vi "(Old Driver) Block Write Iterator.vi"(8 "error in (no error)":errorcluster, 9 "Iterations (1000)":i32=110, 10 "Channel Count":i32, 11 "VMIC-5565":T1) -> (0 "error out":errorcluster, 1 "Histogram Graph":T2(graph), 2 "Metrics":T3 {"Transfer Rate" format="%.2pB/s"; "Duration Std. Dev." format="%.0f µs"; "Duration Average" format="%.0f µs"}, 3 "VMIC-5565 out":T1)   [LabVIEW 2016]
uses:
  Controls/Throughput Metrics.ctl
  <instrlib>/GE 5565 PIORC/Public/DMA Interrupt/GE5565 DMA Write Interrupt (U8) Cluster.vi
  <instrlib>/GE 5565 PIORC/GE 5565 PIORC.lvlib
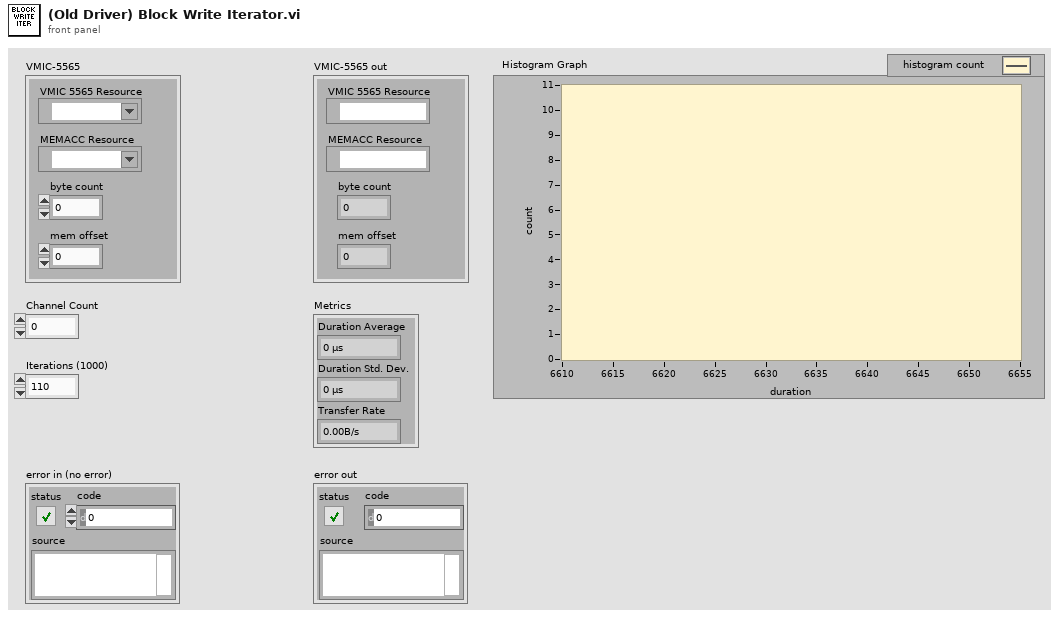
[diagram p1: front panel]
types:
  T1 = cluster{"VMIC 5565 Resource":refnum<visa-resource-name>, "MEMACC Resource":refnum<visa-resource-name>, "byte count":u32, "mem offset":u32}
  T2 = cluster{"X Values":dbl[], "Histogram: h(x)":i32[]}
  T3 = typedef "Throughput Metrics.ctl" = cluster{"Duration Average":u32, "Duration Std. Dev.":u32, "Transfer Rate":dbl}
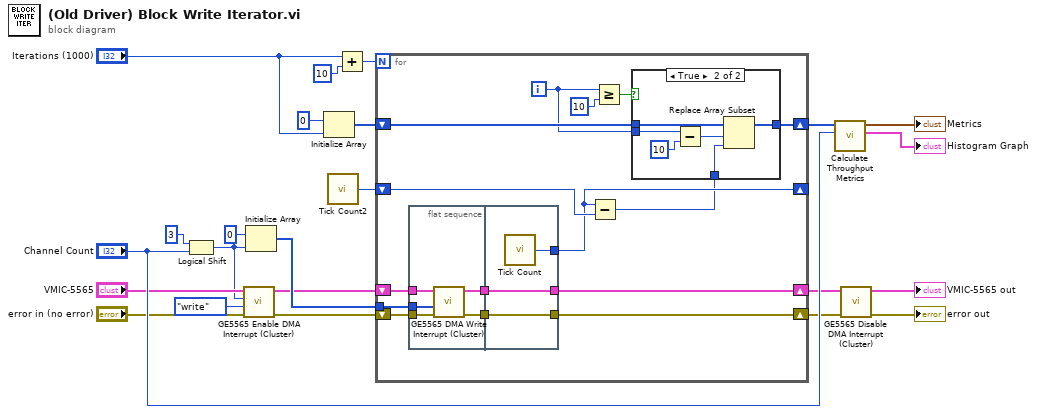
[diagram p0: block diagram]
diagram:
  n1 = Logical Shift(y=i16 3, x="Channel Count") -> (x << y=w5:i32)
  n2 = call <instrlib>:"GE5565 Enable DMA Interrupt (Cluster).vi"("error in (no error)"="error in (no error)", "operation (read)"=enum16{"read", "write"}."write", "transfer size (1024 bytes)"=w5, "VMIC reference in"="VMIC-5565") -> ("error out"=w6:errorcluster, "VMIC reference out"=w7:T1)  [unwired: 2 in]
  n3 = Initialize Array(u8 0 ("element"), w5) -> (w11:u8[])
  n4 = Initialize Array(u32 0 ("x-y"), "Iterations (1000)") -> (w17:u32[])
  n5 = call "Tick Count2"() -> ("Tick Count(uSec)"=w21:u32)
  n6 = Add(x="Iterations (1000)", y=10) -> (x+y=w23:i32)
  n7 = for {
    N: w23 -> [_]
    shift-right: [w31] -> _
    shift-left: w21 -> [w32]
    shift-right: [w34] -> w4
    shift-left: w7 -> [w38]
    shift-right: [w33] -> w3
    shift-left: w6 -> [w37]
    shift-right: [w29] -> w16
    shift-left: w17 -> [w30]
    tunnel: w11 -> [w24]
    i -> [w27]
    n8 = flat-sequence {
      tunnel: w38 -> [w47]
      tunnel: w37 -> [w49]
      tunnel: [w50] -> w36
      tunnel: [w48] -> w25
      tunnel: w24 -> [w46]
      tunnel: [w53] -> w34
      tunnel: w36 -> [w52]
      tunnel: [w52] -> w33
      tunnel: [w51] -> w31
      tunnel: w25 -> [w53]
      frame #0 {
        n9 = call-poly <instrlib>:"GE5565 DMA Write Interrupt (Cluster).vi"("error in (no error)"=w49, "buffer"=w46, "VMIC reference in"=w47) -> ("error out"=w50:errorcluster, "VMIC reference out"=w48:T1)  [unwired: 7 in]
      }
      frame #1 {
        n10 = call "Tick Count"() -> ("Tick Count(uSec)"=w51:u32)
      }
    }
    n11 = Subtract(x=w31, y=w32) -> (x-y=w26:u32)
    n12 = Greater Or Equal?(x=w27, y=10) -> (x >= y?=w28:bool)
    n13 = case shown="True" w28 {
      tunnel: w30 -> [w39 w45]
      tunnel: [w39 w44] -> w29
      tunnel: w27 -> [_ w43]
      tunnel: w26 -> [_ w40]
      frame False {
      }
      frame True {
        n14 = Subtract(x=w43, y=10) -> (x-y=w41:i32)
        n15 = Replace Array Subset(array=w45, new element=w40, index=w41) -> (w44:u32[])
      }
    }
  }
  n16 = call "Calculate Throughput Metrics.vi"("Channel Count"="Channel Count", "Durations"=w16) -> ("Histogram Graph"=→"Histogram Graph":T2, "Metrics"=→"Metrics":T3)  [unwired: 8 in]
  n17 = call <instrlib>:"GE5565 Disable DMA Interrupt (Cluster).vi"("error in (no error)"=w3, "VMIC reference in"=w4) -> ("error out"=→"error out":errorcluster, "VMIC reference out"=→"VMIC-5565 out":T1)  [unwired: 4 in]
